vi "Config-Read Key (string 1D).vi"(0 "configuration file path":path, 2 "section":string="General", 7 "key":string[](array[string]), 9 "default":string, 11 "error in (no error)":errorcluster) -> (4 "file path":path, 8 "found?":bool, 10 "values":string[](array[string]), 15 "error out":errorcluster)   [LabVIEW 2020]
uses:
  <vilib>/Utility/config.llb/Read Key (String).vi
  <vilib>/Utility/config.llb/NI_LVConfig.lvlib
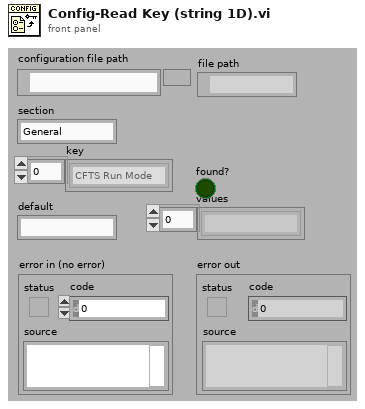
[diagram p1: front panel]
types:
  T1 = typedef "NI_LVConfig.lvlib/Config Data RefNum.ctl" = refnum<k1>
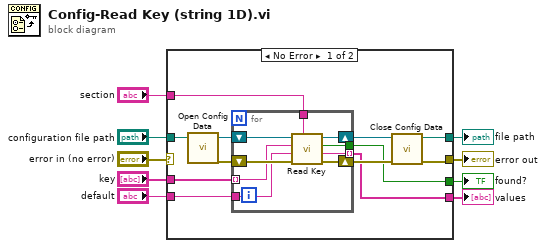
[diagram p0: block diagram]
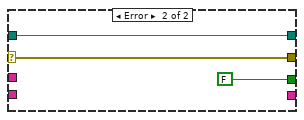
[diagram p2: hidden frame]
diagram:
  n1 = case shown="No Error" "error in (no error)" {
    selector: "error in (no error)" -> [_ w33]
    tunnel: [w19 w33] -> w9
    tunnel: [w10 _] -> w7
    tunnel: "default" -> [w16 _]
    tunnel: "key" -> [w15 _]
    tunnel: "section" -> [w11 _]
    tunnel: "configuration file path" -> [w14 w32]
    tunnel: [w13 w32] -> w2
    tunnel: [w12 FALSE ("found?")] -> w1
    frame No Error {
      n2 = call <vilib>:"Open Config Data.vi"("configuration file path"=w14) -> ("error out"=w21:errorcluster, "refnum"=w20:T1)  [unwired: 8 in, 1 out]
      n3 = for {
        tunnel: w16 -> [w26]
        tunnel: w15 -> [w25] mode=indexing
        tunnel: [w24] -> w12
        shift-right: [w28] -> w18
        shift-left: w21 -> [w30]
        shift-right: [w27] -> w17
        shift-left: w20 -> [w29]
        tunnel: [w23] -> w10 mode=indexing
        tunnel: w11 -> [w22]
        n4 = call-poly <vilib>:"Read Key.vi"("section"=w22, "error in (no error)"=w30, "default value"=w26, "key"=w25, "refnum"=w29) -> ("error out"=w28:errorcluster, "value"=w23:string, "found?"=w24:bool, "refnum out"=w27:T1)  [unwired: 3 in]
      }
      n5 = call <vilib>:"Close Config Data.vi"("error in (no error)"=w18, "refnum"=w17) -> ("error out"=w19:errorcluster, "file path"=w13:path)  [unwired: 8 in]
    }
    frame Error {
    }
  }
  "error out" <- w9
  "values" <- w7
  "file path" <- w2
  "found?" <- w1
